vi "Write Cluster.vi"(8 "error in (no error)":errorcluster, 10 "States":T1, 11 "NewTestTactic in":refnum<class "NewTestTactic.lvclass">) -> (0 "error out":errorcluster, 3 "NewTestTactic out":refnum<class "NewTestTactic.lvclass">)   [LabVIEW 2022 SP3, in "NewTestTactic.lvclass"]
uses:
  NewTestTactic.lvclass
  NewTestTactic.lvclass/NewTestTactic.ctl
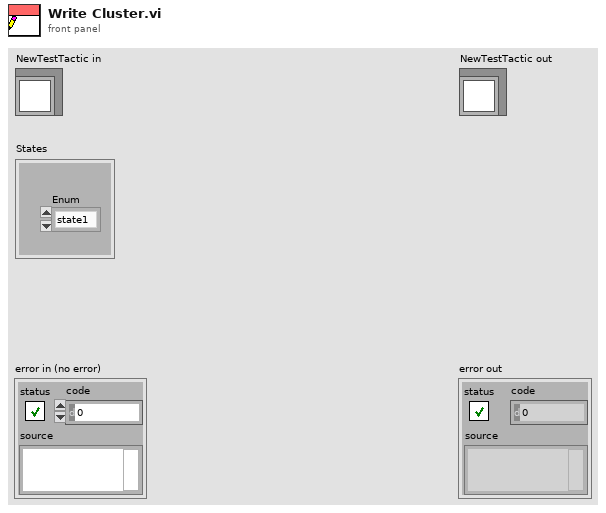
[diagram p1: front panel]
types:
  T1 = cluster{"Enum":enum16{"state1", "ebo", "ebo2", "bo3"}}
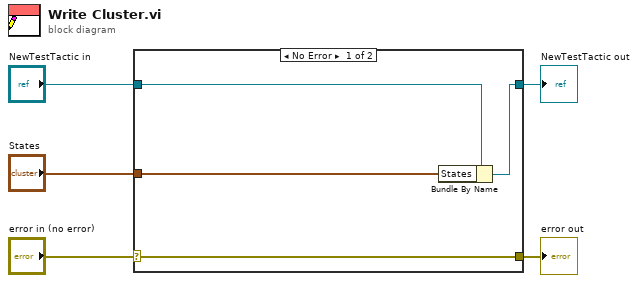
[diagram p0: block diagram]
diagram:
  n1 = case shown="No Error" "error in (no error)" {
    selector: "error in (no error)" -> [w9 w10]
    tunnel: [w9 w10] -> w4
    tunnel: [w7 w11] -> w2
    tunnel: "NewTestTactic in" -> [w8 w11]
    tunnel: "States" -> [w6 _]
    frame No Error {
      n2 = Bundle By Name(cluster=w8, "States"=w6) -> (w7:refnum<class "NewTestTactic.lvclass">)
    }
    frame Error {
    }
  }
  "error out" <- w4
  "NewTestTactic out" <- w2
